vi "Write Test Group Manager.vi"(8 "error in (no error)":errorcluster, 10 "Test Group Manager":refnum<data-value>, 11 "Measurement Interface in":refnum<class "Measurement Interface.lvclass">) -> (0 "error out":errorcluster, 3 "Measurement Interface out":refnum<class "Measurement Interface.lvclass">)   [LabVIEW 2016, in "Measurement Interface.lvlib" / "Measurement Interface.lvclass"]
uses:
  Measurement Interface.lvclass
  Plugins/Test Group Manager.lvlibp/Test Group Manager.lvclass
  Measurement Interface.lvclass/Measurement Interface.ctl
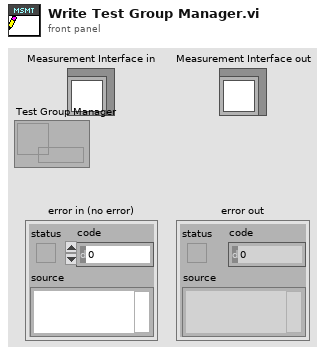
[diagram p1: front panel]
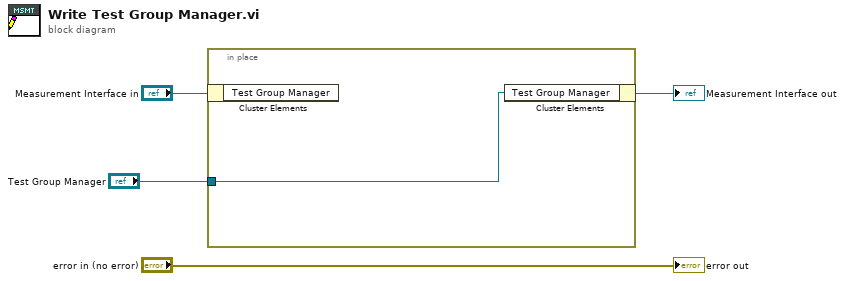
[diagram p0: block diagram]
diagram:
  n1 = in-place {
    in-place-border: "Test Group Manager" -> [w5]
    n2 = in-place-cluster #1("Measurement Interface in") -> ()  [unwired: 1 out]
    n3 = in-place-cluster #1("Test Group Manager"=w5) -> (→"Measurement Interface out":refnum<class "Measurement Interface.lvclass">)
  }
  "error out" <- "error in (no error)"
